vi "ConvertRowAndColumn.vi"(11 "String":string) -> (2 "Column":i32, 3 "Row":i32)   [LabVIEW 2013]
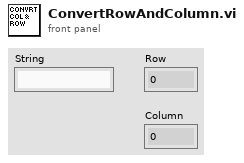
[diagram p1: front panel]
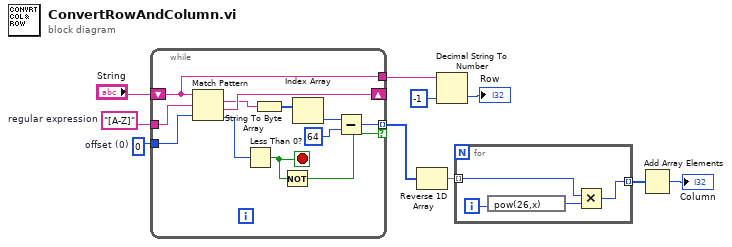
[diagram p0: block diagram]
diagram:
  w2 = "[A-Z]"  # regular expression
  w3 = 0  # offset (0)
  n1 = while {
    tunnel: w2 -> [w22]
    shift-right: [w21] -> _
    shift-left: "String" -> [w18]
    tunnel: w3 -> [w19]
    tunnel: [w18] -> w8
    tunnel: [w15] -> w4 mode=indexing if=w11
    stop <- w12 stop-if-true
    n2 = Match Pattern(string=w18, regular expression=w22, offset (0)=w19) -> (match substring=w17:string, after substring=w21:string, offset past match=w20:i32)  [unwired: 1 out]
    n3 = Less Than 0?(x=w20) -> (x < 0?=w12:bool)
    n4 = String To Byte Array(string=w17) -> (unsigned byte array=w16:u8[])
    n5 = Not(x=w12) -> (.not. x?=w11:bool)
    n6 = Index Array(array=w16) -> (element=w14:u8)  [unwired: 1 in]
    n7 = Subtract(x=w14, y=u8 64) -> (x-y=w15:u8)
  }
  n8 = Reverse 1D Array(array=w4) -> (reversed array=w7:u8[])
  n9 = Decimal String To Number(string=w8, default (0L)=-1 ("default (0 I32)")) -> (number=→"Row":i32)  [unwired: 1 in, 1 out]
  n10 = for {
    tunnel: w7 -> [w24] mode=indexing
    tunnel: [w23] -> w5 mode=indexing
    i -> [w26]
    n11 = expression code="pow(26,x)"(w26) -> (w25:i32)
    n12 = Multiply(x=w24, y=w25) -> (x*y=w23:i32)
  }
  n13 = Add Array Elements(numeric array=w5) -> (sum=→"Column":i32)
